vi "Login Flir-Ax8.vi"(3 "Password":string, 4 "User Name":string, 5 "IP":string) -> (0 "Error":errorcluster, 1 "Image Request":string, 2 "Client Handle":T1)   [LabVIEW 2016]
uses:
  <vilib>/httpClient/ClientHandle.ctl
  <vilib>/httpClient/POSTBuffer.vi
  <vilib>/httpClient/LabVIEWHTTPClient.lvlib
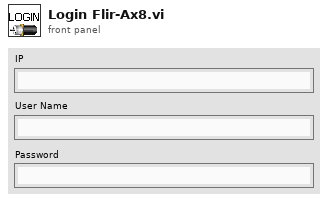
[diagram p1: front panel]
types:
  T1 = typedef "LabVIEWHTTPClient.lvlib/ClientHandle.ctl" = refnum<k1>
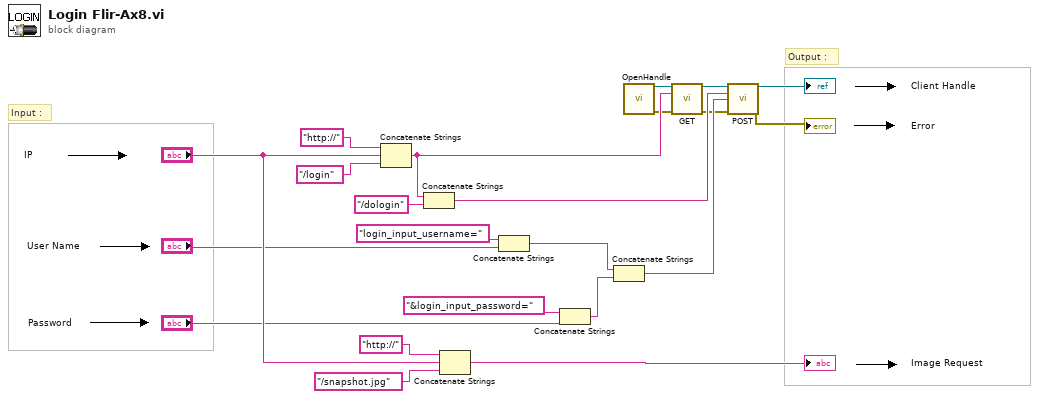
[diagram p0: block diagram]
diagram:
  # "Output :"
  # "Input :"
  n1 = Concatenate Strings ("add")("http://" ("string"), "IP", "/login" ("string")) -> (w18:string)
  n2 = Concatenate Strings ("add")(w18, "/dologin" ("url")) -> (w16:string)
  n3 = Concatenate Strings ("add")("http://" ("string"), "IP", "/snapshot.jpg" ("string")) -> (→"Image Request":string)
  n4 = Concatenate Strings ("add")("login_input_username=" ("string"), "User Name") -> (w13:string)
  n5 = Concatenate Strings ("add")("&login_input_password=" ("string"), "Password") -> (w12:string)
  n6 = Concatenate Strings ("add")(w13, w12) -> (w11:string)
  n7 = call <vilib>:"OpenHandle.vi"() -> ("client handle out"=w19:T1, "error out"=w6:errorcluster)  [unwired: 14 in]
  n8 = call <vilib>:"GET.vi"("client handle"=w19, "url"=w18, "error in (no error)"=w6) -> ("client handle out"=w17:T1, "error out"=w5:errorcluster)  [unwired: 9 in, 2 out]
  n9 = call-poly <vilib>:"POST.vi"("client handle"=w17, "url"=w16, "buffer"=w11, "error in (no error)"=w5) -> ("client handle out"=→"Client Handle":T1, "error out"=→"Error":errorcluster)  [unwired: 8 in, 2 out]
